vi "Labview File_Digital_Signal_Assignment.vi"() -> ()   [LabVIEW 2018]
uses:
  <vilib>/Analysis/3filter.llb/Filter Passband Type.ctl
  <vilib>/Analysis/2dsp.llb/Real FFT.vi
  <vilib>/Waveform/WDTFileIO.llb/Read Waveform from File.vi
  <vilib>/Analysis/3filter.llb/IIR Filter (DBL).vi
  <vilib>/Analysis/3filter.llb/Butterworth Filter (DBL).vi
  <vilib>/Analysis/NI_AALPro.lvlib
  <vilib>/Analysis/NI_AALBase.lvlib
  <vilib>/measure/NI_MABase.lvlib
panel:
  out "lowpass filter output 9":waveform(dbl)(graph)
  out "IIR filter time domain 3":waveform(dbl)(graph)
  out "binary 7":waveform(dbl)(graph)
  out "rectifier output 6":waveform(dbl)(graph)
  out "demodulation 5":waveform(dbl)(graph)
  out "sin waveform 4":waveform(dbl)(graph)
  out "IIR filter frequency domain 3":waveform(dbl)(graph)
  out "given signal 1":dbl[](graph)
  out "Given signal in Frequency domain 2":waveform(dbl)(graph)
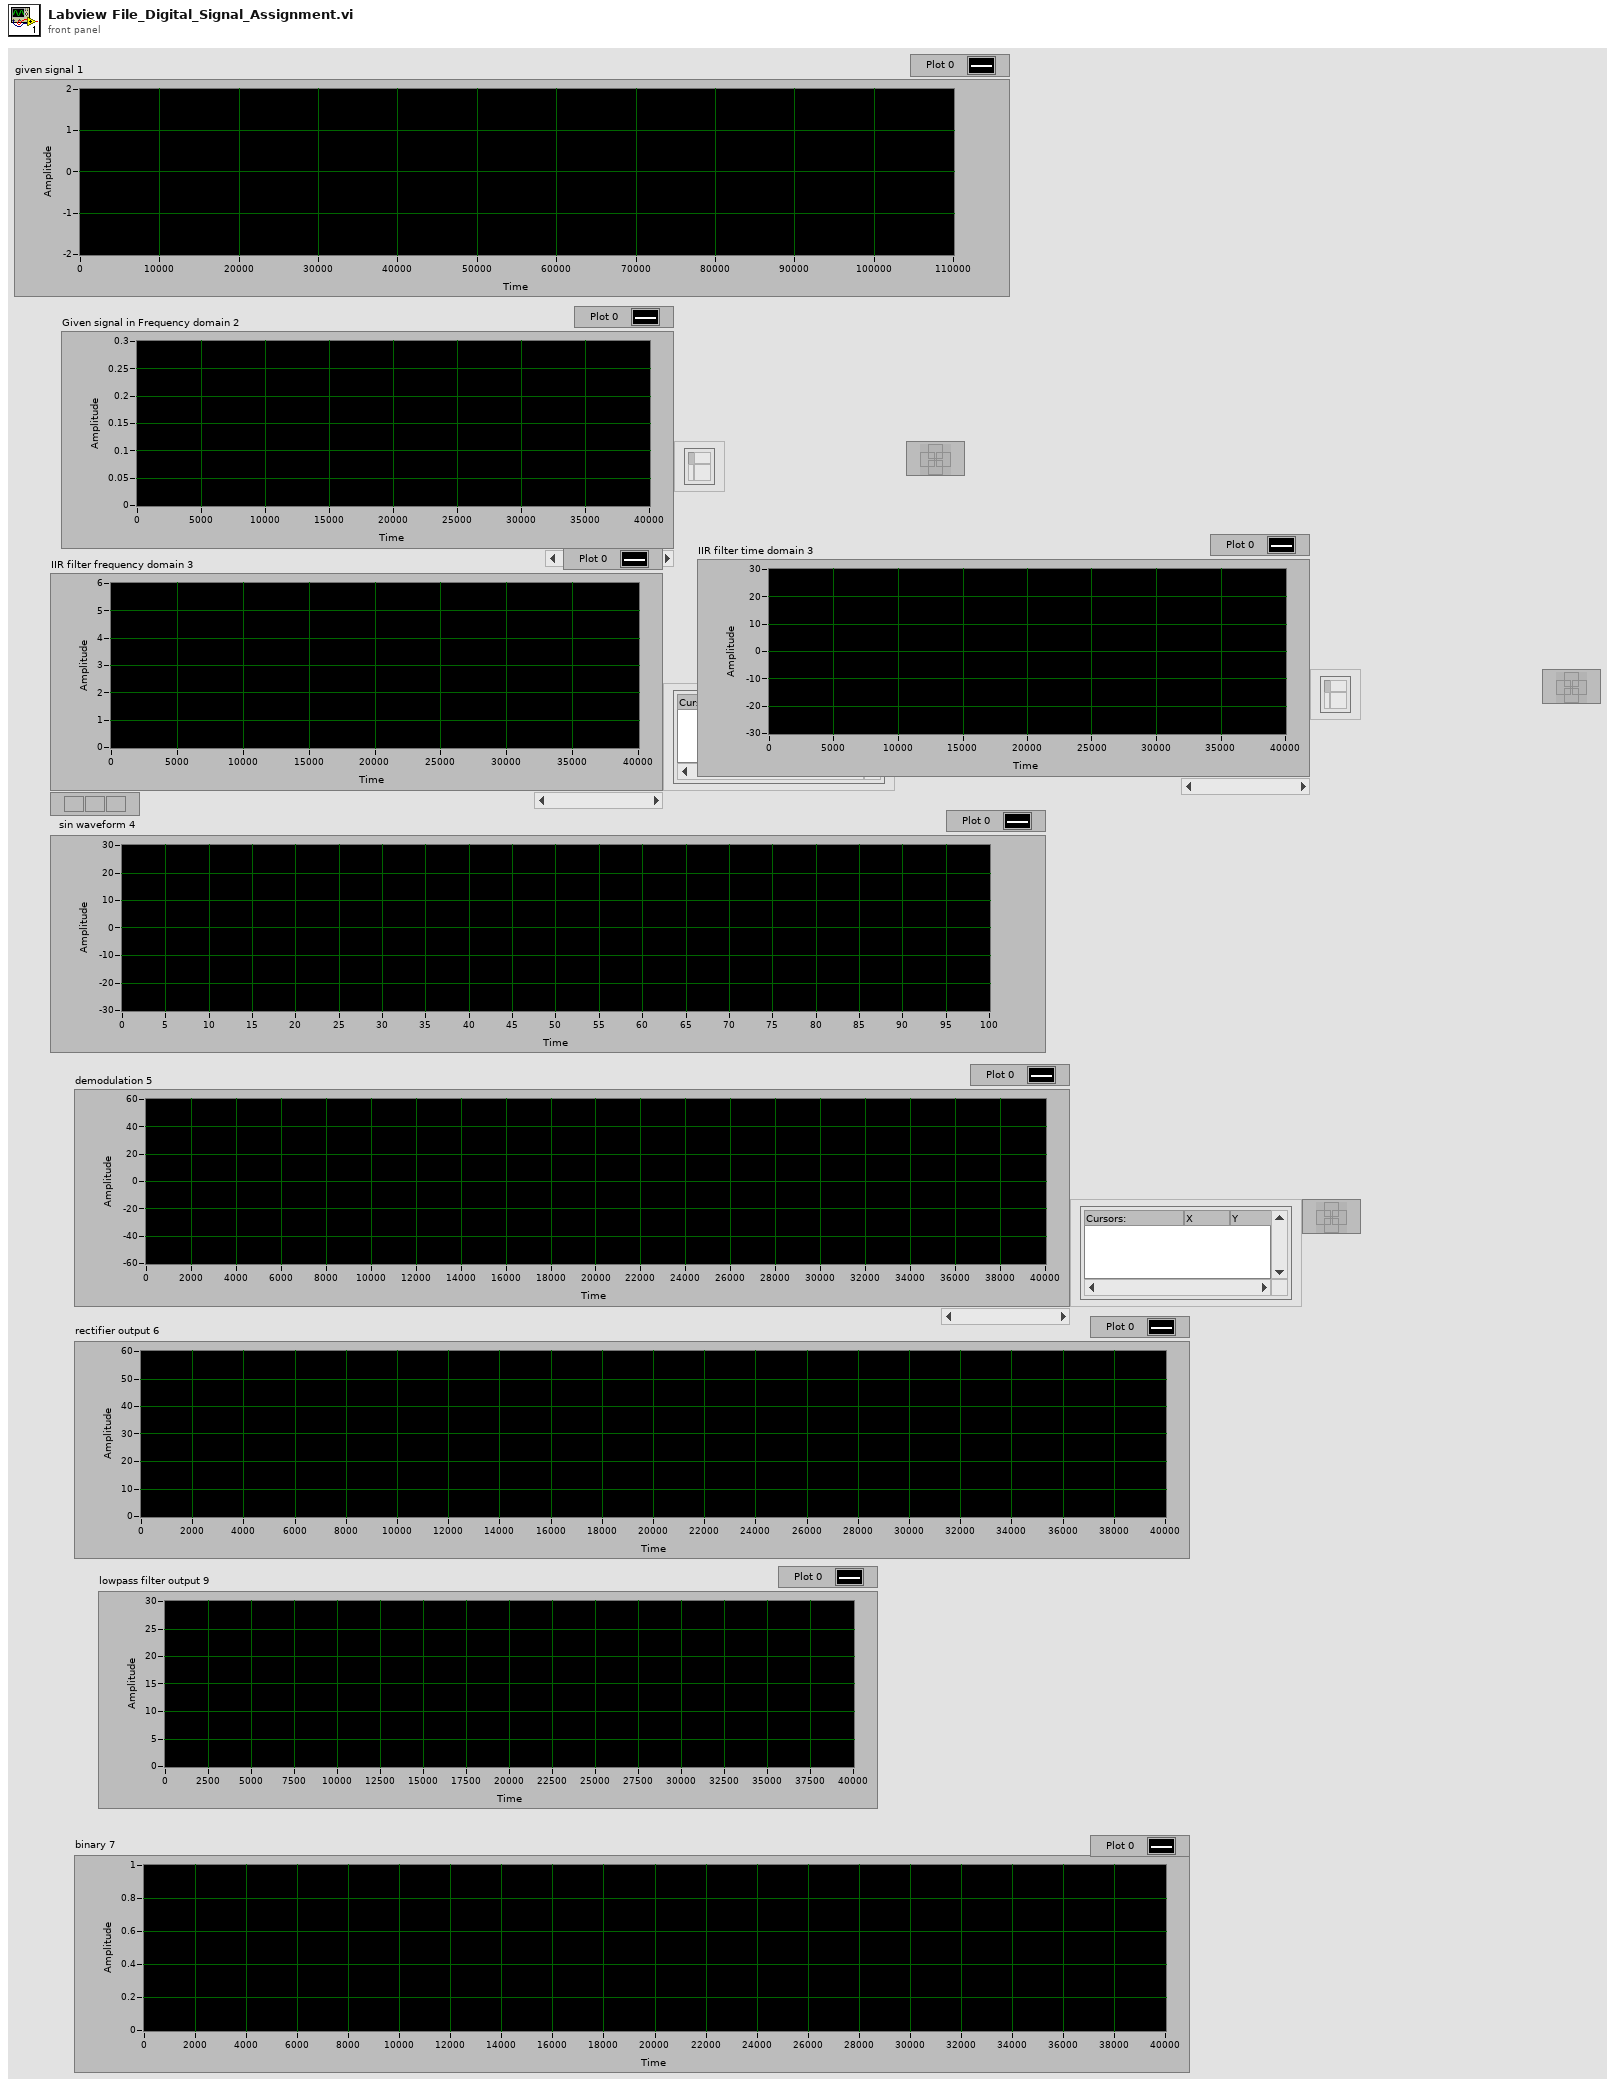
[diagram p1: front panel]
types:
  T1 = typedef "NI_AALBase.lvlib/Filter Passband Type.ctl" = enum32{"Lowpass", "Highpass", "Bandpass", "Bandstop"}
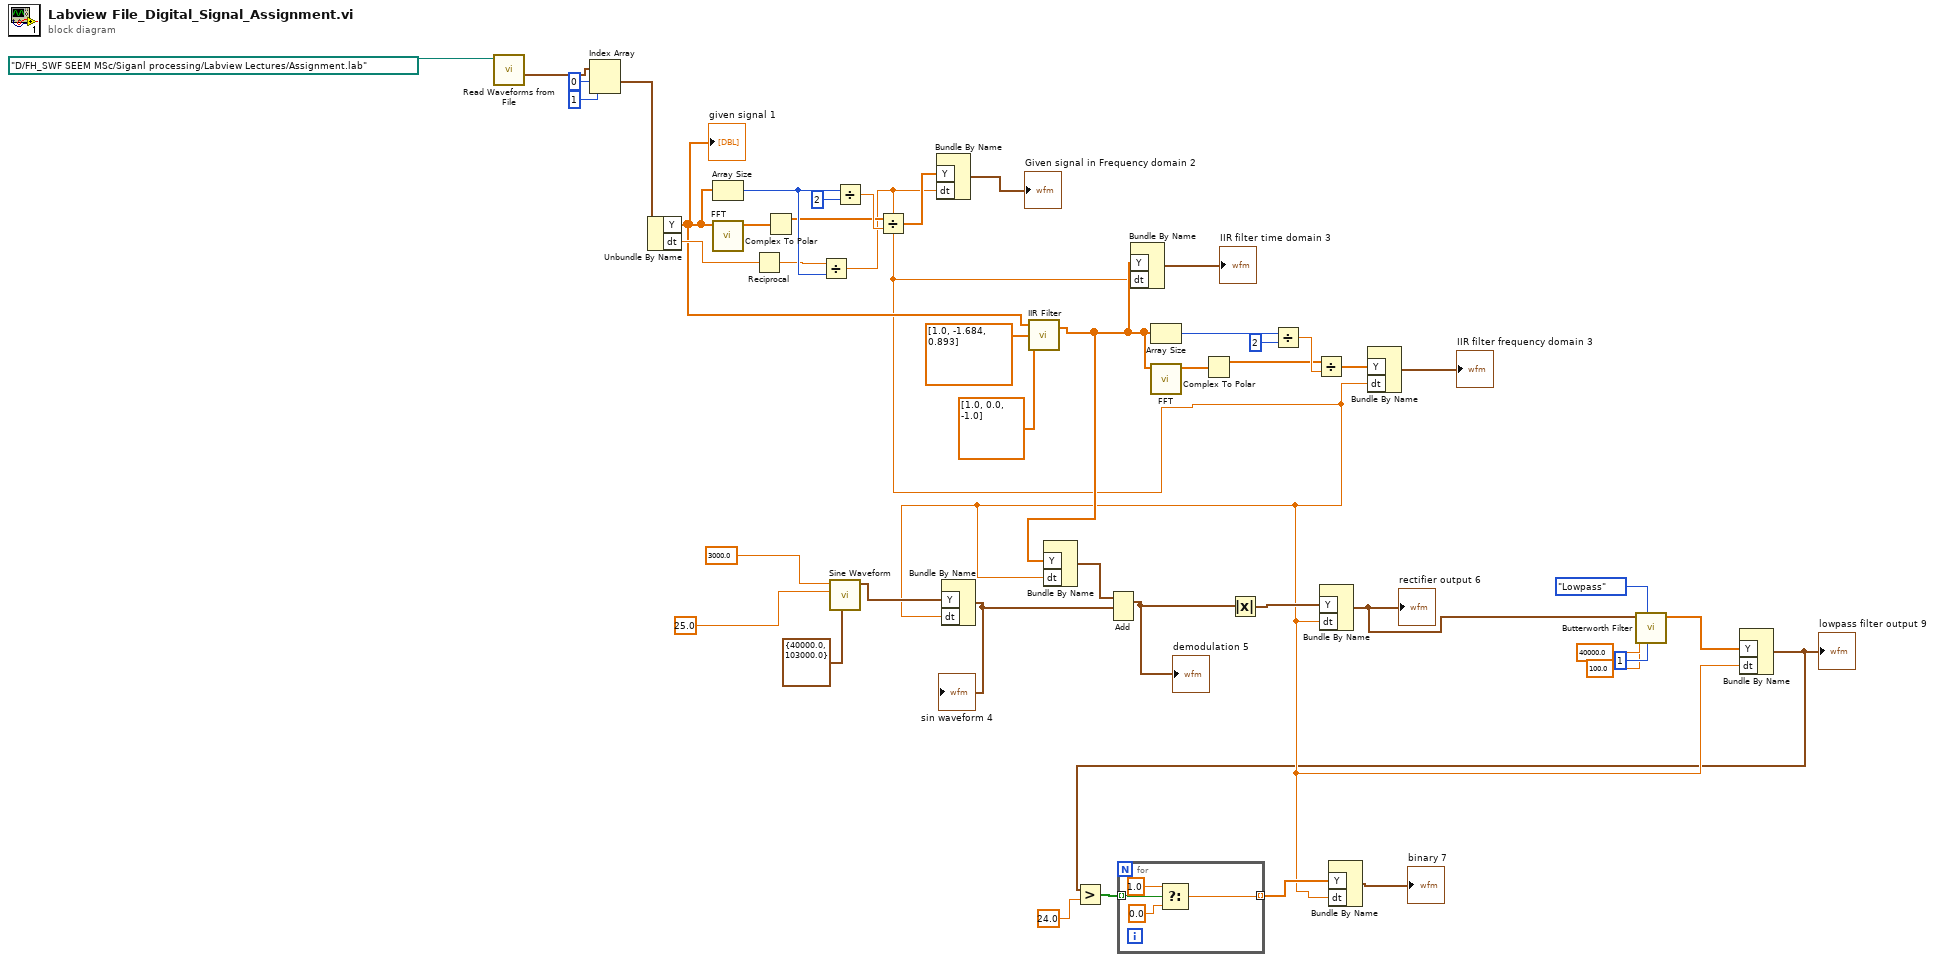
[diagram p0: block diagram]
diagram:
  n1 = call-poly <vilib>:"Read Waveforms from File.vi"("file path (dialog if empty)"=path "D:/FH_SWF SEEM MSc/Siganl processing/Labview Lectures/Assignment.lab") -> ("all waveforms in record"=w43:waveform(dbl)[])  [unwired: 5 in, 3 out]
  n2 = Index Array(array=w43, index #1=0 ("index"), index #2=1 ("index")) -> (element #1=w35:waveform(dbl))  [unwired: 1 out]
  n3 = Unbundle By Name(w35) -> ("Y"=w14:dbl[], "dt"=w41:dbl)
  "given signal 1" <- w14
  n4 = Array Size(array=w14) -> (size(s)=w40:i32)
  n5 = call-poly <vilib>:"FFT.vi"("X"=w14) -> ("FFT {X}"=w39:cdb[])  [unwired: 9 in, 1 out]
  n6 = Reciprocal(x=w41) -> (1/x=w34:dbl)
  n7 = Complex To Polar(r * e^(i*theta)=w39) -> (r=w37:dbl[])  [unwired: 1 out]
  n8 = Divide(x=w34, y=w40) -> (x/y=w7:dbl)
  n9 = call <vilib>:"Sine Waveform.vi"("sampling info"=cluster{"Fs":dbl, "#s":dbl} {"Fs"=40000.0, "#s"=103000.0}, "amplitude"=25.0, "frequency"=3000.0 ("Sin Wave frequency")) -> ("signal out"=w23:waveform(dbl))  [unwired: 7 in, 1 out]
  n10 = Divide(x=w40, y=2) -> (x/y=w38:dbl)
  n11 = Divide(x=w37, y=w38) -> (x/y=w36:dbl[])
  n12 = Bundle By Name("Y"=w36, "dt"=w7) -> (→"Given signal in Frequency domain 2":waveform(dbl))  [unwired: 1 in]
  n13 = Bundle By Name("Y"=w23, "dt"=w7) -> (w22:waveform(dbl))  [unwired: 1 in]
  "sin waveform 4" <- w22
  n14 = call-poly <vilib>:"IIR Filter.vi"("Forward Coefficients"=dbl[] [1.0, 0.0, -1.0], "Reverse Coefficients"=dbl[] [1.0, -1.684, 0.893], "X"=w14) -> ("Filtered X"=w11:dbl[])  [unwired: 1 in, 1 out]
  n15 = Bundle By Name("Y"=w11, "dt"=w7) -> (w16:waveform(dbl))  [unwired: 1 in]
  n16 = Add(1:w22, 2:w16) -> (0:w18:waveform(dbl))  [unwired: 1 in, 1 out]
  "demodulation 5" <- w18
  n17 = Bundle By Name("Y"=w11, "dt"=w7) -> (→"IIR filter time domain 3":waveform(dbl))  [unwired: 1 in]
  n18 = Array Size(array=w11) -> (size(s)=w31:i32)
  n19 = call-poly <vilib>:"FFT.vi"("X"=w11) -> ("FFT {X}"=w30:cdb[])  [unwired: 9 in, 1 out]
  n20 = Complex To Polar(r * e^(i*theta)=w30) -> (r=w28:dbl[])  [unwired: 1 out]
  n21 = Absolute Value(x=w18) -> (abs(x)=w13:waveform(dbl))
  n22 = Divide(x=w31, y=2) -> (x/y=w29:dbl)
  n23 = Divide(x=w28, y=w29) -> (x/y=w27:dbl[])
  n24 = Bundle By Name("Y"=w13, "dt"=w7) -> (w6:waveform(dbl))  [unwired: 1 in]
  "rectifier output 6" <- w6
  n25 = Bundle By Name("Y"=w27, "dt"=w7) -> (→"IIR filter frequency domain 3":waveform(dbl))  [unwired: 1 in]
  n26 = call-poly <vilib>:"Butterworth Filter.vi"("order"=1, "filter type"=Filter_Passband_Type."Lowpass", "low cutoff freq: fl"=100.0, "sampling freq: fs"=40000.0, "X"=w6) -> ("Filtered X"=w9:dbl[])  [unwired: 3 in, 1 out]
  n27 = Bundle By Name("Y"=w9, "dt"=w7) -> (w3:waveform(dbl))  [unwired: 1 in]
  "lowpass filter output 9" <- w3
  n28 = Greater?(x=w3, y=24.0) -> (0:w20:bool[])
  n29 = for {
    tunnel: w20 -> [w50] mode=indexing
    tunnel: [w47] -> w19 mode=indexing
    n30 = Select(t=1.0, s=w50, f=0.0) -> (s? t:f=w47:dbl)
  }
  n31 = Bundle By Name("Y"=w19, "dt"=w7) -> (→"binary 7":waveform(dbl))  [unwired: 1 in]
